vi "Test Helper Loop No Error Restarting.vi"(8 "error in (no error)":errorcluster, 11 "Helper Loop Test in":refnum<class "Helper Loop Test.lvclass">) -> (0 "error out":errorcluster, 3 "Helper Loop Test out":refnum<class "Helper Loop Test.lvclass">)   [LabVIEW 2020, in "Helper Loop Test.lvclass"]
uses:
  Helper Loop Test.lvclass
  C:/Program Files (x86)/National Instruments/LabVIEW 2020/vi.lib/Asteme/LUnit/Test Case.lvclass
  Framework/Process/Public/Lifecycle/Lifecycle State.ctl
  Mock Error Handler/Mock Error Handler.lvclass
  C:/Users/anton/Documents/GitHub/Triarc-Framework/source/Framework/Error Handler Interface/Error Handler Interface.lvclass
  Mock Process/Mock Process.lvclass
  C:/Users/anton/Documents/GitHub/Triarc-Framework/source/Framework/Process/Process.lvclass
  Framework/Process/Process.lvclass/Process.ctl
  <vilib>/Asteme/LUnit/Test Case.lvclass/Test Case.ctl
  <vilib>/Asteme/LUnit/LUnit Assertion Result.lvclass/LUnit Assertion Result.ctl
  Framework/Process/Protected/Messaging/Enqueue Message.vi
  Framework/Process/Public/Lifecycle/Get Lifecycle State.vi
  Framework/Process/Private/SubVIs/Wait for finish.vi
  Framework/Process/Private/SubVIs/Set Lifecycle State.vi
  <vilib>/Asteme/LUnit/Palette/Pass If.vi
  <vilib>/Asteme/LUnit/Set Assertion Type.vi
  <vilib>/Asteme/LUnit/Palette/Pass.vi
  <vilib>/Asteme/LUnit/Palette/Fail.vi
  <vilib>/Utility/error.llb/Clear Errors.vi
  <vilib>/Asteme/LUnit/LUnit Write Assertion Type.vi
  <vilib>/Asteme/LUnit/Add test result.vi
  <vilib>/Asteme/LUnit/LUnit Write Passed.vi
  <vilib>/Asteme/LUnit/LUnit Get Test Case.vi
  <vilib>/Asteme/LUnit/Assertion Result/LUnit Get Test Name.vi
  <vilib>/Asteme/LUnit/LUnit Write Message.vi
  <vilib>/Asteme/LUnit/LUnit Write Description.vi
  <vilib>/Asteme/LUnit/Read Test Case Name.vi
  <vilib>/Utility/error.llb/Error Cluster From Error Code.vi
  <vilib>/Asteme/LUnit/LUnit Assertion Result.lvclass
  Framework/Process/Process.lvclass
  <vilib>/Asteme/LUnit/Test Case.lvclass
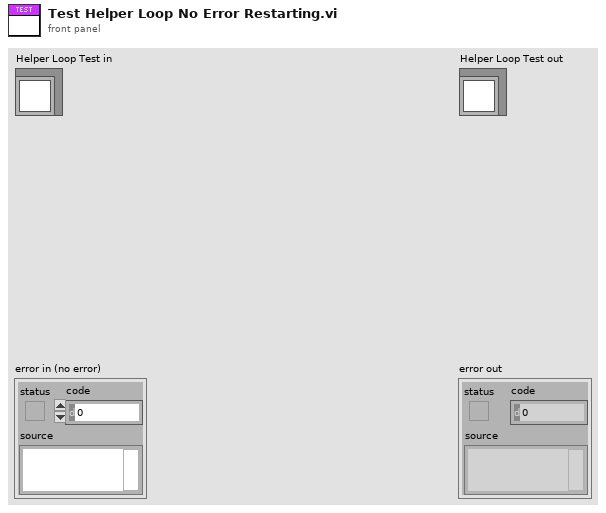
[diagram p1: front panel]
types:
  T1 = typedef "Process.lvclass/Lifecycle State.ctl" = enum16{"Uninitialized", "Initialized", "Started", "Running", "Stopped", "Finished"}
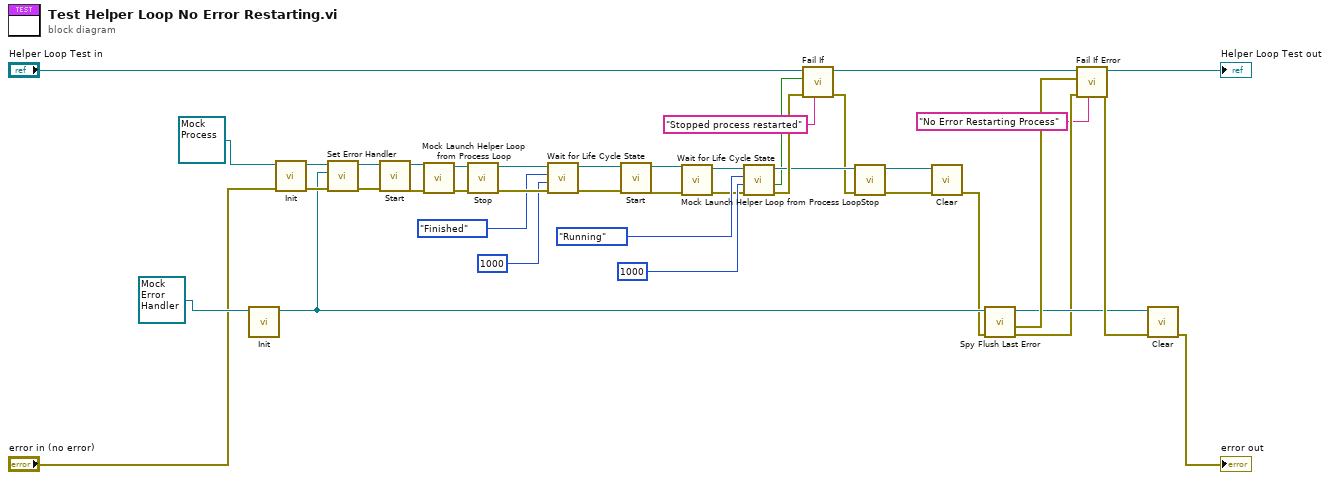
[diagram p0: block diagram]
diagram:
  n1 = call-dynamic "Init.vi"("Mock Error Handler In"=refnum<class "Mock Error Handler.lvclass"> refnum ("Mock Error Handler.lvclass")) -> ("Mock Error Handler Out"=w18:refnum<class "Mock Error Handler.lvclass">)  [unwired: 9 in, 1 out]
  n2 = call-dynamic "Init.vi"("error in (no error)"="error in (no error)", "Mock Process In"=refnum<class "Mock Process.lvclass"> refnum) -> ("error out"=w40:errorcluster, "Mock Process Out"=w23:refnum<class "Mock Process.lvclass">)  [unwired: 8 in]
  n3 = call "Set Error Handler.vi"("error in (no error)"=w40, "Error Handler"=w18, "Process In"=w23) -> ("error out"=w24:errorcluster, "Process Out"=w22:refnum<class "Mock Process.lvclass">)  [unwired: 7 in]
  n4 = call "Start.vi"("error in (no error)"=w24, "Process In"=w22) -> ("error out"=w41:errorcluster, "Process Out"=w9:refnum<class "Mock Process.lvclass">)  [unwired: 8 in]
  n5 = call "Mock Launch Helper Loop from Process Loop.vi"("error in (no error)"=w41, "Mock Process in"=w9) -> ("error out"=w10:errorcluster, "Mock Process out"=w8:refnum<class "Mock Process.lvclass">)  [unwired: 8 in]
  n6 = call "Stop.vi"("error in (no error)"=w10, "Process In"=w8) -> ("error out"=w36:errorcluster, "Process Out"=w34:refnum<class "Mock Process.lvclass">)  [unwired: 7 in, 1 out]
  n7 = call "Wait for Life Cycle State.vi"("error in (no error)"=w36, "timeout in ms (-1)"=1000, "Lifecycle State"=Lifecycle_State."Finished", "Process In"=w34) -> ("error out"=w35:errorcluster, "Process Out"=w33:refnum<class "Mock Process.lvclass">)  [unwired: 5 in, 1 out]
  n8 = call "Start.vi"("error in (no error)"=w35, "Process In"=w33) -> ("error out"=w39:errorcluster, "Process Out"=w6:refnum<class "Mock Process.lvclass">)  [unwired: 8 in]
  n9 = call "Mock Launch Helper Loop from Process Loop.vi"("error in (no error)"=w39, "Mock Process in"=w6) -> ("error out"=w7:errorcluster, "Mock Process out"=w5:refnum<class "Mock Process.lvclass">)  [unwired: 8 in]
  n10 = call "Wait for Life Cycle State.vi"("error in (no error)"=w7, "timeout in ms (-1)"=1000, "Lifecycle State"=Lifecycle_State."Running", "Process In"=w5) -> ("error out"=w30:errorcluster, "timed out?"=w25:bool, "Process Out"=w29:refnum<class "Mock Process.lvclass">)  [unwired: 5 in]
  n11 = call <vilib>:"Fail If.vi"("Description"="Stopped process restarted", "error in (no error)"=w30, "Fail?"=w25, "Test Case In"="Helper Loop Test in") -> ("error out"=w26:errorcluster, "Test Case Out"=w20:refnum<class "Helper Loop Test.lvclass">)  [unwired: 6 in]
  n12 = call "Stop.vi"("error in (no error)"=w26, "Process In"=w29) -> ("error out"=w37:errorcluster, "Process Out"=w38:refnum<class "Mock Process.lvclass">)  [unwired: 7 in, 1 out]
  n13 = call-dynamic "Clear.vi"("error in (no error)"=w37, "Mock Process In"=w38) -> ("error out"=w15:errorcluster)  [unwired: 9 in]
  n14 = call "Spy Flush Last Error.vi"("error in (no error)"=w15, "Mock Error Handler In"=w18) -> ("error out"=w14:errorcluster, "Error"=w19:errorcluster, "Mock Error Handler Out"=w16:refnum<class "Mock Error Handler.lvclass">)  [unwired: 7 in]
  n15 = call <vilib>:"Fail If Error.vi"("Description"="No Error Restarting Process", "error in (no error)"=w14, "Assert error"=w19, "Test Case In"=w20) -> ("error out"=w17:errorcluster, "Test Case Out"=→"Helper Loop Test out":refnum<class "Helper Loop Test.lvclass">)  [unwired: 6 in]
  n16 = call-dynamic "Clear.vi"("error in (no error)"=w17, "Mock Process In"=w16) -> ("error out"=→"error out":errorcluster)  [unwired: 9 in]
